vi "reset.vi"(8 "error in (no error)":errorcluster, 11 "IP address":string="192.168.10.17") -> (0 "error out":errorcluster)   [LabVIEW 2017]
panel:
  out "Out":u8 format="%.0x"
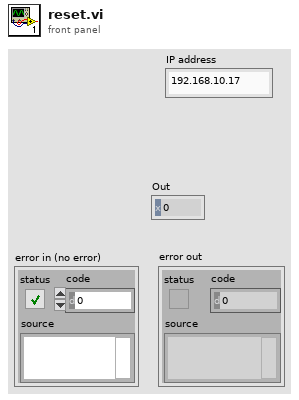
[diagram p1: front panel]
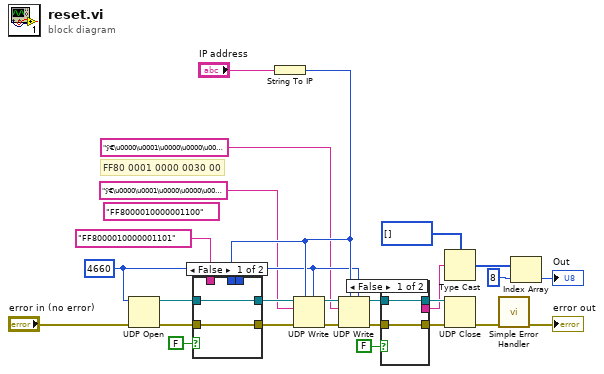
[diagram p0: block diagram]
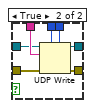
[diagram p2: hidden frame]
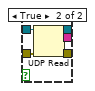
[diagram p3: hidden frame]
diagram:
  (unwired) "FF8000010000001100" ("data in")
  w8 = u16 4660 ("UDP port")
  # "FF80 0001 0000 0030 00"
  n1 = UDP Open(8:"error in (no error)", 11:w8) -> (port=w5:refnum<k16>, 0:w7:errorcluster)  [unwired: 3 in, 1 out]
  n2 = String To IP(1:"IP address") -> (0:w9:u32)
  n3 = case shown="False" FALSE {
    tunnel: "FF8000010000001101" ("data in") -> [_ w35]
    tunnel: w9 -> [_ w34]
    tunnel: w8 -> [_ w33]
    tunnel: w7 -> [w28 w32]
    tunnel: [w28 w31] -> w6
    tunnel: w5 -> [w27 w30]
    tunnel: [w27 w29] -> w4
    frame False {
    }
    frame True {
      n4 = UDP Write(address=w34, port or service name=w33, connection ID=w30, data in=w35, 8:w32) -> (error out=w31:errorcluster, 3:w29:refnum<k16>)  [unwired: 1 in]
    }
  }
  n5 = UDP Write(address=w9, port or service name=w8, connection ID=w4, data in="ÿ€\u0000\u0001\u0000\u0000\u0000\u0011\u0000" ("字符串"), 8:w6) -> (error out=w13:errorcluster, 3:w12:refnum<k16>)  [unwired: 1 in]
  n6 = UDP Write(address=w9, port or service name=w8, connection ID=w12, data in="ÿ€\u0000\u0001\u0000\u0000\u0000\u0010\u0001" ("字符串"), 8:w13) -> (error out=w23:errorcluster, 3:w25:refnum<k16>)  [unwired: 1 in]
  n7 = case shown="False" FALSE {
    tunnel: w25 -> [w37 w42]
    tunnel: [w37 w41] -> w24
    tunnel: w23 -> [w36 w40]
    tunnel: [w36 w39] -> w22
    tunnel: [_ w38] -> w21
    frame False {
    }
    frame True {
      n8 = UDP Read(connection ID=w42, 8:w40) -> (data out=w38:string, error out=w39:errorcluster, 3:w41:refnum<k16>)  [unwired: 1 in, 3 out]
    }
  }
  n9 = Type Cast(type=u8[] [], x=w21) -> (*(type *) &x=w19:u8[])
  n10 = UDP Close(connection ID=w24, 8:w22) -> (error out=w26:errorcluster)  [unwired: 1 out]
  n11 = call <vilib>:"Simple Error Handler.vi"("error in (no error)"=w26) -> ("error out"=→"error out":errorcluster)  [unwired: 4 in, 4 out]
  n12 = Index Array(array=w19, index=8) -> (element=→"Out":u8)
